vi "WAPIAerSend.vi"(8 "error in (no error)":errorcluster, 11 "lpsCmd":string) -> (0 "error out":errorcluster)   [LabVIEW 2009]
uses:
  win50032.dll
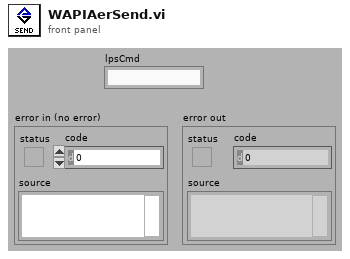
[diagram p1: front panel]
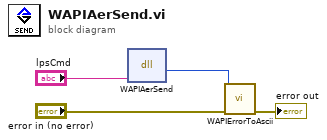
[diagram p0: block diagram]
diagram:
  n1 = dll-call lib="win50032.dll" fn="WAPIAerSend"("lpsCmd"="lpsCmd") -> ("return type"=w4:u32)  [unwired: 4 in, 2 out]
  n2 = call "WAPIErrorToAscii.vi"("error in (no error)"="error in (no error)", "error"=w4) -> ("error out"=→"error out":errorcluster)  [unwired: 8 in, 1 out]
